vi "Talon Position Control.vi"(0 "CAN Talon SRX Ref":T2={"DeviceStatus"={"status"=FALSE, "code"=0, "source"=""}, "Type"=enum."PWM", "PWM"={"PWM Channel"=enum."Invalid", "DeadBand"={"Name"="", "maxPositivePwm"=0, "minPositivePwm"=0, "centerPwm"=0, "maxNegativePwm"=0, "minNegativePwm"=0, "angularRange"=0}}, "CAN"={"Device Number"=0, "Control Mode"=enum."Percent VBus", "Semaphore"=refnum, "Max Vout"=12.0, "TalonSRX Control Mode"=enum."Percent VBus"}, "Invert"=FALSE}, 1 "Post-Shaft Gear Ratio":dbl=1.0, 5 "Joystick":dbl, 7 "Move to Target?":bool, 9 "Target Degrees":dbl, 11 "error in (no error)":errorcluster, 12 "PID Parameters":T8) -> (4 "CAN Talon SRX Ref":T2={"DeviceStatus"={"status"=FALSE, "code"=0, "source"=""}, "Type"=enum."PWM", "PWM"={"PWM Channel"=enum."PWM 1", "DeadBand"={"Name"="", "maxPositivePwm"=0, "minPositivePwm"=0, "centerPwm"=0, "maxNegativePwm"=0, "minNegativePwm"=0, "angularRange"=0}}, "CAN"={"Device Number"=0, "Control Mode"=enum."Percent VBus", "Semaphore"=refnum, "Max Vout"=12.0, "TalonSRX Control Mode"=enum."Percent VBus"}, "Invert"=FALSE}, 6 "Control Mode":T1, 10 "Encoder Count Target":dbl, 15 "error out":errorcluster)   [LabVIEW 2015]
uses:
  <vilib>/Rock Robotics/WPI/MotorControl/WPI_MotorControlDeviceRef.ctl
  <vilib>/Rock Robotics/WPI/MotorControl/WPI_MotorControlType.ctl
  <vilib>/Rock Robotics/SystemInterfaces/DIO/FPGA_DIOPWMChannel.ctl
  <vilib>/Rock Robotics/WPI/PWM/WPI_PWMDeadband.ctl
  <vilib>/Rock Robotics/WPI/CAN/Jaguar/SubVIs/WPI_CANJaguar_ControlMode.ctl
  <vilib>/Rock Robotics/WPI/CAN/TalonSRX/WPI_CANTalonSRX_APIControlMode.ctl
  <vilib>/Rock Robotics/WPI/CAN/TalonSRX/WPI_CANTalonSRX_APIFeedbackSelect.ctl
  <vilib>/Rock Robotics/WPI/CAN/TalonSRX/WPI_CANTalonSRX_Params.ctl
panel:
  out "SensorPos (rotations)":dbl
  out "Motor output Plot":cluster{"Applied Throttle":dbl}(graph)
  out "Target Position (rotations)":dbl
  out "SensorRPM Velocity RPM":dbl
  out "Applied Output":dbl
  out "Position Closed Loop Plots":cluster{dbl, "Sensor Velocity":dbl}(graph)
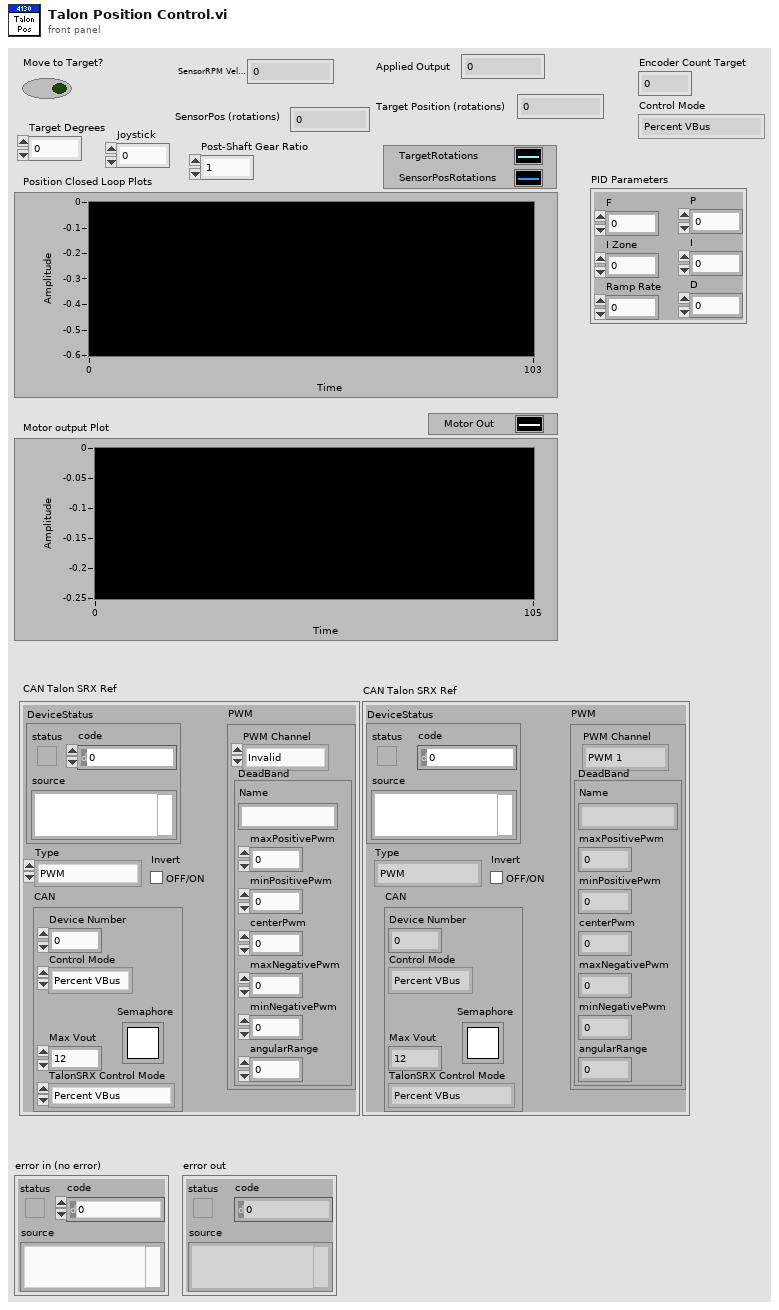
[diagram p1: front panel]
types:
  T1 = typedef "WPI_CANTalonSRX_APIControlMode.ctl" = enum8{"Percent VBus", "Speed", "Position", "Slave", "Unchanged / Invalid", "Voltage Compensation", "Current", "Motion Profile"}
  T2 = typedef "WPI_MotorControlDeviceRef.ctl" = cluster{"DeviceStatus":errorcluster, "Type":T3, "PWM":cluster{"PWM Channel":T4, "DeadBand":T5}, "CAN":cluster{"Device Number":u8, "Control Mode":T6, "Semaphore":T7, "Max Vout":dbl, "TalonSRX Control Mode":T1}, "Invert":bool}
  T3 = typedef "WPI_MotorControlType.ctl" = enum16{"PWM", "CAN", "CANTalonSRX"}
  T4 = typedef "FPGA_DIOPWMChannel.ctl" = enum8{"PWM 0", "PWM 1", "PWM 2", "PWM 3", "PWM 4", "PWM 5", "PWM 6", "PWM 7", "PWM 8", "PWM 9", "PWM MXP 0", "PWM MXP 1", "PWM MXP 2", "PWM MXP 3", "PWM MXP 4", "PWM MXP 5", "PWM MXP 6", "PWM MXP 7", "PWM MXP 8", "PWM MXP 9", "Invalid"}
  T5 = typedef "WPI_PWMDeadband.ctl" = cluster{"Name":string, "maxPositivePwm":i32, "minPositivePwm":i32, "centerPwm":i32, "maxNegativePwm":i32, "minNegativePwm":i32, "angularRange":u16}
  T6 = typedef "WPI_CANJaguar_ControlMode.ctl" = enum8{"Percent VBus", "Current", "Speed", "Position", "Voltage"}
  T7 = typedef "Semaphore RefNum" = refnum<k1>
  T8 = cluster{"F":dbl, "I Zone":dbl, "Ramp Rate":dbl, "P":dbl, "I":dbl, "D":dbl}
  T9 = typedef "WPI_CANTalonSRX_APIFeedbackSelect.ctl" = enum16{"Digital Quadrature Encoder", "Analog Potentiometer", "Analog Encoder", "Count on Quad-A (Rising-Edge)", "Count on Quad-A (Falling-Edge)", "CTR Magnetic Enc (Absolute)", "CTR Magnetic Enc (Relative)", "Pulse Width"}
  T10 = typedef "WPI_CANTalonSRX_GlobalStatus.ctl" = cluster{"Applied Throttle":dbl, "Module Enabled":bool, "CAN Error":errorcluster, "Closed Loop Error":dbl, "Forward Limit Switch Closed":bool, "Reverse Limit Switch Closed":bool, "Sensor Position":dbl, "Sensor Velocity":dbl, "Current":dbl, "Sticky Fault - Over Temp":bool, "Sticky Fault - Under Voltage":bool, "Sticky Fault - Forward Limit":bool, "Sticky Fault - Reverse Limit":bool, "Sticky Fault - Forward Soft Limit":bool, "Sticky Fault - Reverse Soft Limit":bool, "Brake is Enabled":bool, "Encoder Position":dbl, "Encoder Velocity":dbl, "Encoder Index Count":dbl, "Encoder A Pin State":bool, "Encoder B Pin State":bool, "Encoder Index Pin State":bool, "Analog In":dbl, "Analog In Velocity":dbl, "Temperature (C)":dbl, "Battery Voltage":dbl, "Control 5 Is Supported":bool, "Current Profile Slot Select":dbl, "Pos Div 8":bool, "Vel Div 4":bool, "Pulse Width Position":i32, "Pulse Width Velocity":i32, "Pulse Width Rise To Rise (us)":i32, "Pulse Width Rise To Fall (us)":i32, "Mot Prof Active Is Under Run":bool, "Mot Prof Active Has Under Run":bool, "Mot Prof Active Is Last":bool, "Mot Prof Active Velocity Only":bool, "Mot Prof Active Is Valid":bool, "Mot Prof Buffer Is Full":bool, "Mot Prof Active Profile Slot Select":i32, "Mot Prof NextID":i32, "Mot Prof Count":i32, "Mot Prof Active Velocity":dbl, "Mot Prof Active Position":dbl, "Mot Prof Output Enable":i32}
  T11 = typedef "WPI_CANTalonSRX_Params.ctl" = u8
  T12 = cluster{"Target Degrees":dbl, "Sensor Position":dbl}
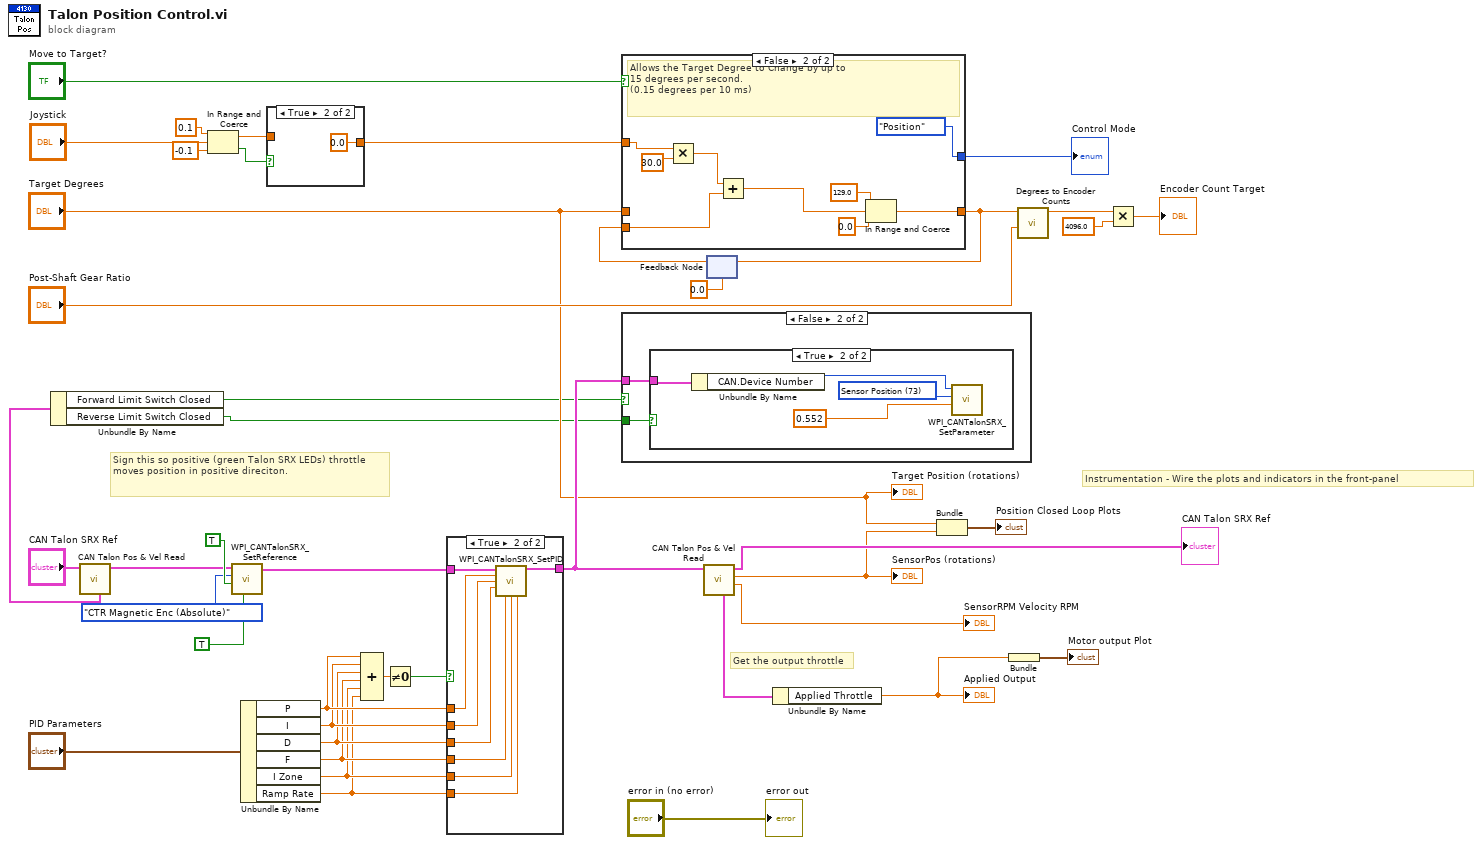
[diagram p0: block diagram]
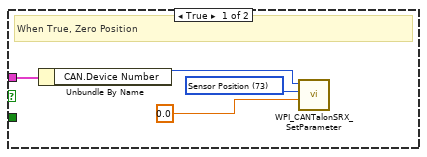
[diagram p4: hidden frame]
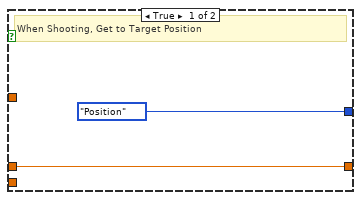
[diagram p6: hidden frame]
diagram:
  # "Sign this so positive (green Talon SRX LEDs) throttle moves position in positive direciton."
  # "Instrumentation - Wire the plots and indicators in the front-panel"
  # "Get the output throttle"
  n1 = call "CAN Talon Pos & Vel Read.vi"("CAN Talon SRX Ref"="CAN Talon SRX Ref") -> ("CAN Talon SRX Ref"=w13:T2, "Talon SRX Status"=w12:T10)  [unwired: 6 in, 3 out]
  n2 = Unbundle By Name(w12) -> ("Forward Limit Switch Closed"=w11:bool, "Reverse Limit Switch Closed"=w1:bool)
  n3 = In Range and Coerce(upper limit=0.1, x="Joystick", lower limit=-0.1) -> (coerced(x)=w5:dbl, In Range?=w6:bool)
  n4 = call <vilib>:"WPI_CANTalonSRX_SetReference.vi"("Reverse Closed-Loop Output"=TRUE, "Reverse Feedback Sensor"=TRUE, "Feedback Reference"=WPI_CANTalonSRX_APIFeedbackSelect."CTR Magnetic Enc (Absolute)", "CAN Talon SRX Ref"=w13) -> ("CAN Talon SRX Ref"=w36:T2)  [unwired: 6 in, 1 out]
  n5 = Unbundle By Name("PID Parameters") -> ("P"=w21:dbl, "I"=w20:dbl, "D"=w19:dbl, "F"=w18:dbl, "I Zone"=w17:dbl, "Ramp Rate"=w16:dbl)
  n6 = case shown="True" w6 {
    tunnel: w5 -> [w43 _]
    tunnel: [w43 0.0 ("upper limit")] -> w4
    frame False {
    }
    frame True {
    }
  }
  n7 = Compound Arithmetic op=ADD(w21, w20, w19, w18, w17, w16) -> (w15:dbl)
  n8 = Not Equal To 0?(x=w15) -> (x != 0?=w14:bool)
  n9 = case shown="True" w14 {
    tunnel: w36 -> [w45 w53]
    tunnel: [w45 w52] -> w33
    tunnel: w21 -> [_ w51]
    tunnel: w20 -> [_ w50]
    tunnel: w19 -> [_ w49]
    tunnel: w18 -> [_ w48]
    tunnel: w17 -> [_ w47]
    tunnel: w16 -> [_ w46]
    frame False {
    }
    frame True {
      n10 = call <vilib>:"WPI_CANTalonSRX_SetPID.vi"("CAN Talon SRX Ref"=w53, "P"=w51, "I"=w50, "D"=w49, "F"=w48, "I Zone"=w47, "Ramp Rate"=w46) -> ("CAN Talon SRX Ref"=w52:T2)  [unwired: 7 in, 1 out]
    }
  }
  "CAN Talon SRX Ref" <- w33
  n11 = case shown="False" w11 {
    tunnel: w33 -> [w54 w59]
    tunnel: w1 -> [_ w58]
    frame True {
      w57 = T11 73 items=["Slot 0 - P"=1, "Slot 0 - I"=2, "Slot 0 - D"=3, "Slot 0 - F"=4, "Slot 0 - I Zone"=5, "Slot 0 - Ramp Rate"=6, "Slot 1 - P"=11, "Slot 1 - I"=12, "Slot 1 - D"=13, "Slot 1 - F"=14, "Slot 1 - I Zone"=15, "Slot 1 - Ramp Rate"=16, "Soft Limit - Forward"=21, "Soft Limit - Reverse"=22, "Soft Limit - Forward Enable"=23, "Soft Limit - Reverse Enable"=24, "On Boot - Brake Mode"=31, "On Boot - Limit Normally Closed - Forward"=32, "On Boot - Limit Normally Closed - Reverse"=33, "On Boot - Limit Disabled - Forward"=34, "On Boot - Limit Disabled - Reverse"=35, "Fault - Over Temp"=41, "Fault - Under Voltage"=42, "Fault - Forward Limit"=43, "Fault - Reverse Limit"=44, "Fault - Hardware Failure"=45, "Fault - Forward Soft Limit"=46, "Fault - Reverse Soft Limit"=47, "Sticky Fault - Over Temp"=48, "Sticky Fault - Under Voltage"=49, "Sticky Fault - Forward Limit"=50, "Sticky Fault - Reverse Limit"=51, "Sticky Fault - Forward Soft Limit"=52, "Sticky Fault - Reverse Soft Limit"=53, "Applied Throttle"=61, "Closed-Loop Error"=62, "Select Feedback Device"=63, "Reverse Closed-Loop Output"=64, "Mode Select"=65, "Profile Slot Select"=66, "Ramp Throttle"=67, "Reverse Feedback Sensor"=68, "Limit Switch Enabled"=69, "Limit Switch Closed - Forward"=70, "Limit Switch Closed - Reverse"=71, "Sensor Position"=73, "Sensor Velocity"=74, "Current"=75, "Brake is Enabled"=76, "Encoder Position"=77, "Encoder Velocity"=78, "Encoder Index Rise Events"=79, "Encoder A Pin State"=80, "Encoder B Pin State"=81, "Encoder Index Pin State"=82, "Analog In with Overflow"=83, "Analog In Velocity"=84, "Temperature"=85, "Battery Voltage"=86, "Reset Count"=87, "Reset Flags"=88, "Firmware Version"=89, "Settings Changed"=90, "Quad Filter Enable"=91, "Ignore Disable Broadcast"=92, "I Accumulator"=93, "Status 1 Frame Rate Ms"=94, "Status 2 Frame Rate Ms"=95, "Status 3 Frame Rate Ms"=96, "Status 4 Frame Rate Ms"=97, "Status 6 Frame Rate Ms"=98, "Status 7 Frame Rate Ms"=99, "Enable Index Pin Clear Position"=100, "Peak Positive Output"=104, "Nominal Positive Output"=105, "Peak Negative Output"=106, "Nominal Negative Output"=107, "Quad Index Pin Polarity"=108, "Status 8 Frame Rate Ms"=109, "Allow Position Overflow"=110, "Slot 0 - Allowable Closed-Loop Error"=111, "Number Potentiometer Turns"=112, "Encoder Codes Per Rev"=113, "Pulse Width Decoded Position"=114, "Analog Position"=115, "Voltage Compensation Rate (V/s)"=116, "Slot 1 - Allowable Closed-Loop Error"=117, "Motion Profile Has Underrun Err"=119] ("Parameter")
      # "When True, Zero Position"
      n12 = Unbundle By Name(w54) -> ("CAN.Device Number"=w56:u8)
      n13 = call <vilib>:"WPI_CANTalonSRX_SetParameter.vi"("Value"=0.0, "Parameter"=w57, "Device ID (0)"=w56) -> ()  [unwired: 7 in, 2 out]
    }
    frame False {
      n14 = case shown="True" w58 {
        tunnel: w59 -> [_ w60]
        frame False {
        }
        frame True {
          w63 = T11 73 items=["Slot 0 - P"=1, "Slot 0 - I"=2, "Slot 0 - D"=3, "Slot 0 - F"=4, "Slot 0 - I Zone"=5, "Slot 0 - Ramp Rate"=6, "Slot 1 - P"=11, "Slot 1 - I"=12, "Slot 1 - D"=13, "Slot 1 - F"=14, "Slot 1 - I Zone"=15, "Slot 1 - Ramp Rate"=16, "Soft Limit - Forward"=21, "Soft Limit - Reverse"=22, "Soft Limit - Forward Enable"=23, "Soft Limit - Reverse Enable"=24, "On Boot - Brake Mode"=31, "On Boot - Limit Normally Closed - Forward"=32, "On Boot - Limit Normally Closed - Reverse"=33, "On Boot - Limit Disabled - Forward"=34, "On Boot - Limit Disabled - Reverse"=35, "Fault - Over Temp"=41, "Fault - Under Voltage"=42, "Fault - Forward Limit"=43, "Fault - Reverse Limit"=44, "Fault - Hardware Failure"=45, "Fault - Forward Soft Limit"=46, "Fault - Reverse Soft Limit"=47, "Sticky Fault - Over Temp"=48, "Sticky Fault - Under Voltage"=49, "Sticky Fault - Forward Limit"=50, "Sticky Fault - Reverse Limit"=51, "Sticky Fault - Forward Soft Limit"=52, "Sticky Fault - Reverse Soft Limit"=53, "Applied Throttle"=61, "Closed-Loop Error"=62, "Select Feedback Device"=63, "Reverse Closed-Loop Output"=64, "Mode Select"=65, "Profile Slot Select"=66, "Ramp Throttle"=67, "Reverse Feedback Sensor"=68, "Limit Switch Enabled"=69, "Limit Switch Closed - Forward"=70, "Limit Switch Closed - Reverse"=71, "Sensor Position"=73, "Sensor Velocity"=74, "Current"=75, "Brake is Enabled"=76, "Encoder Position"=77, "Encoder Velocity"=78, "Encoder Index Rise Events"=79, "Encoder A Pin State"=80, "Encoder B Pin State"=81, "Encoder Index Pin State"=82, "Analog In with Overflow"=83, "Analog In Velocity"=84, "Temperature"=85, "Battery Voltage"=86, "Reset Count"=87, "Reset Flags"=88, "Firmware Version"=89, "Settings Changed"=90, "Quad Filter Enable"=91, "Ignore Disable Broadcast"=92, "I Accumulator"=93, "Status 1 Frame Rate Ms"=94, "Status 2 Frame Rate Ms"=95, "Status 3 Frame Rate Ms"=96, "Status 4 Frame Rate Ms"=97, "Status 6 Frame Rate Ms"=98, "Status 7 Frame Rate Ms"=99, "Enable Index Pin Clear Position"=100, "Peak Positive Output"=104, "Nominal Positive Output"=105, "Peak Negative Output"=106, "Nominal Negative Output"=107, "Quad Index Pin Polarity"=108, "Status 8 Frame Rate Ms"=109, "Allow Position Overflow"=110, "Slot 0 - Allowable Closed-Loop Error"=111, "Number Potentiometer Turns"=112, "Encoder Codes Per Rev"=113, "Pulse Width Decoded Position"=114, "Analog Position"=115, "Voltage Compensation Rate (V/s)"=116, "Slot 1 - Allowable Closed-Loop Error"=117, "Motion Profile Has Underrun Err"=119] ("Parameter")
          n15 = Unbundle By Name(w60) -> ("CAN.Device Number"=w62:u8)
          n16 = call <vilib>:"WPI_CANTalonSRX_SetParameter.vi"("Value"=0.552, "Parameter"=w63, "Device ID (0)"=w62) -> ()  [unwired: 7 in, 2 out]
        }
      }
    }
  }
  n17 = call "CAN Talon Pos & Vel Read.vi"("CAN Talon SRX Ref"=w33) -> ("Sensor Velocity"=→"SensorRPM Velocity RPM":dbl, "Sensor Position"=w31:dbl, "Talon SRX Status"=w30:T10)  [unwired: 6 in, 2 out]
  "SensorPos (rotations)" <- w31
  n18 = feedback #1(0.0 ("Encoder Counts")) -> (w28:dbl)
  n19 = case shown="False" "Move to Target?" {
    tunnel: "Target Degrees" -> [w65 _]
    tunnel: [w65 w68] -> w23
    tunnel: [WPI_CANTalonSRX_APIControlMode."Position" ("Control Mode") WPI_CANTalonSRX_APIControlMode."Position" ("Control Mode")] -> w26
    tunnel: w28 -> [_ w73]
    tunnel: w4 -> [_ w72]
    frame True {
      # "When Shooting, Get to Target Position"
    }
    frame False {
      # "Allows the Target Degree to Change by up to\n15 degrees per second.\n(0.15 degrees per 10 ms)"
      n20 = Multiply(x=w72, y=30.0) -> (x*y=w70:dbl)
      n21 = Add(x=w70, y=w73) -> (x+y=w69:dbl)
      n22 = In Range and Coerce(upper limit=129.0, x=w69, lower limit=0.0) -> (coerced(x)=w68:dbl)  [unwired: 1 out]
    }
  }
  "Control Mode" <- w26
  n23 = feedback-in #1(w23) -> ()
  n24 = Unbundle By Name(w30) -> ("Applied Throttle"=w42:dbl)
  "Applied Output" <- w42
  n25 = Bundle("Target Degrees"="Target Degrees", "Sensor Position"=w31) -> (→"Position Closed Loop Plots":T12)  [unwired: 1 in]
  n26 = Bundle("Applied Throttle"=w42) -> (→"Motor output Plot":cluster{"Applied Throttle":dbl})  [unwired: 1 in]
  n27 = call "Degrees to Encoder Counts.vi"("Post-Shaft Gear Ratio"="Post-Shaft Gear Ratio", "Degrees"=w23) -> ("Encoder Counts"=w22:dbl)  [unwired: 9 in]
  n28 = Multiply(x=w22, y=4096.0) -> (x*y=→"Encoder Count Target":dbl)
  "Target Position (rotations)" <- "Target Degrees"
  "error out" <- "error in (no error)"
